vi "Write Class Type.vi"(8 "error in (no error)":errorcluster, 10 "BC class type":T1 items=["BC"=0, "BC_Steady"=100, "BC_Steady_2D"=120, "BC_Steady_2D_Numeric"=121, "BC_Steady_2D_VIRef"=122, "BC_Evolut"=200, "BC_Evolut_1D"=210, "BC_Evolut_1D_Numeric"=211, "BC_Evolut_1D_VIRef"=212, "BC_Evolut_2D"=220, "BC_Evolut_2D_Numeric"=221, "BC_Evolut_2D_VIRef"=222], 11 "BC.lvclass in":refnum<class "NI_BC.lvclass">) -> (0 "error out":errorcluster, 3 "BC.lvclass out":refnum<class "NI_BC.lvclass">)   [LabVIEW 2020, in "NI_PDE.lvlib" / "NI_BC.lvclass"]
uses:
  <vilib>/gmath/pde.llb/BCClass/NI_BC.lvclass
  <vilib>/gmath/pde.llb/BCClass/Class Type.ctl
  <vilib>/gmath/pde.llb/BCClass/NI_BC.lvclass/NI_BC.ctl
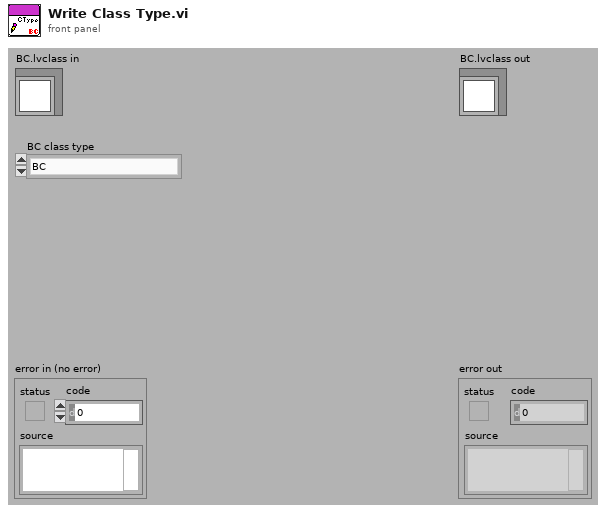
[diagram p1: front panel]
types:
  T1 = typedef "NI_PDE.lvlib/NI_BC.lvclass/Class Type.ctl" = i32
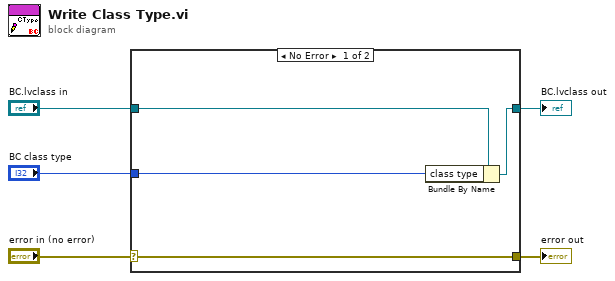
[diagram p0: block diagram]
diagram:
  n1 = case shown="No Error" "error in (no error)" {
    selector: "error in (no error)" -> [w9 w10]
    tunnel: [w9 w10] -> w4
    tunnel: [w7 w11] -> w2
    tunnel: "BC.lvclass in" -> [w8 w11]
    tunnel: "BC class type" -> [w6 _]
    frame No Error {
      n2 = Bundle By Name(cluster=w8, "class type"=w6) -> (w7:refnum<class "NI_BC.lvclass">)
    }
    frame Error {
    }
  }
  "error out" <- w4
  "BC.lvclass out" <- w2
